vi "Random_signal_activity10.vi"() -> ()   [LabVIEW 2025]
panel:
  in  "Loop delay":dbl(knob) scale=0.0..2.0
  out "RandomSignal":dbl(graph)
  in  "Enable":bool
  # "off"
  # "on"
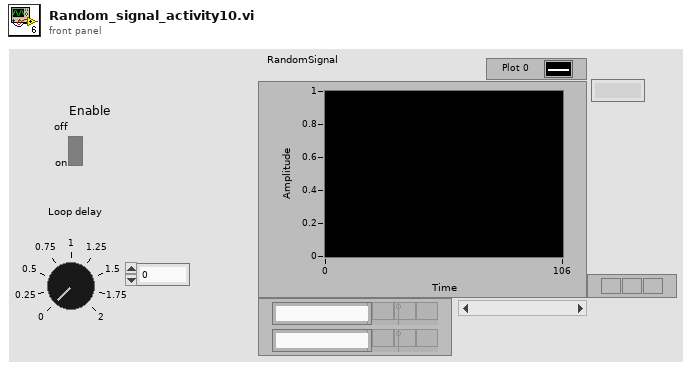
[diagram p1: front panel]
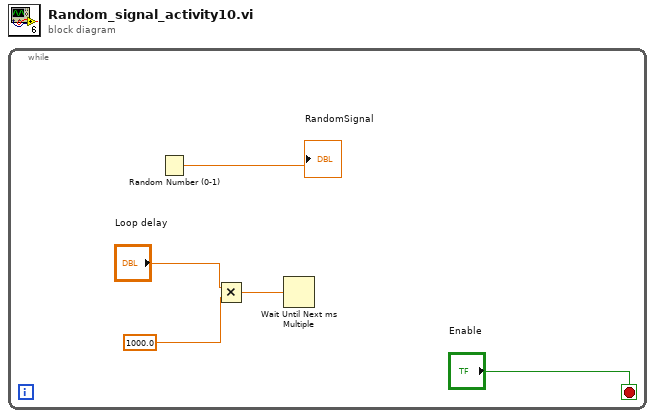
[diagram p0: block diagram]
diagram:
  n1 = while {
    stop <- "Enable" stop-if-true
    n2 = Random Number (0-1)() -> (number: 0 to 1=→"RandomSignal":dbl)
    n3 = Multiply(x="Loop delay", y=1000.0) -> (x*y=w1:dbl)
    n4 = Wait Until Next ms Multiple(millisecond multiple=w1) -> ()  [unwired: 1 out]
  }
